vi "tcp_test.vi"() -> ()   [LabVIEW 2019]
panel:
  out "String 3":string
  in  "Numeric 2":i32=7001
  in  "String 2":string="127.0.0.1"
  in  "String":string
  out "Numeric":dbl
  in  "Boolean":bool
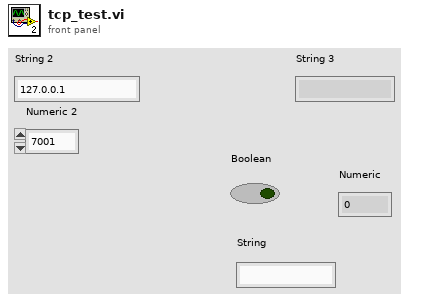
[diagram p1: front panel]
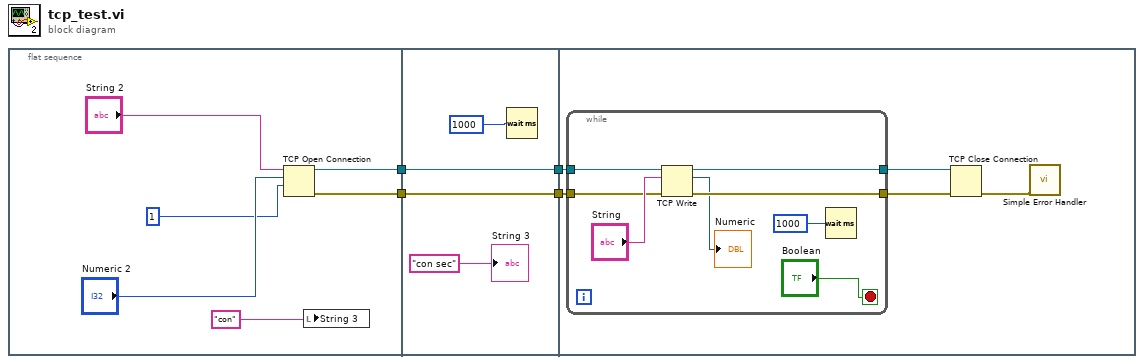
[diagram p0: block diagram]
diagram:
  n1 = flat-sequence {
    tunnel: [w8] -> w2
    tunnel: [w7] -> w1
    tunnel: [w14] -> w4
    tunnel: [w13] -> w3
    tunnel: w2 -> [w14]
    tunnel: w1 -> [w13]
    tunnel: w4 -> [w19]
    tunnel: w3 -> [w18]
    frame #0 {
      n2 = TCP Open Connection(address="String 2", remote port or service name="Numeric 2", timeout ms (60000)=1) -> (connection ID=w8:refnum<k5>, error out=w7:errorcluster)  [unwired: 2 in]
      n3 = local write "String 3"("con") -> ()
    }
    frame #1 {
      n4 = Wait (ms)(milliseconds to wait=1000) -> ()  [unwired: 1 out]
      "String 3" <- "con sec"
    }
    frame #2 {
      n5 = while {
        tunnel: w19 -> [w26]
        tunnel: w18 -> [w21]
        tunnel: [w25] -> w17
        tunnel: [w24] -> w16
        stop <- "Boolean" stop-if-true
        n6 = TCP Write(connection ID=w26, data in="String", error in (no error)=w21) -> (connection ID out=w25:refnum<k5>, bytes written=→"Numeric":i32, error out=w24:errorcluster)  [unwired: 1 in]
        n7 = Wait (ms)(milliseconds to wait=1000) -> ()  [unwired: 1 out]
      }
      n8 = TCP Close Connection(connection ID=w17, error in (no error)=w16) -> (error out=w15:errorcluster)  [unwired: 1 in, 1 out]
      n9 = call <vilib>:"Simple Error Handler.vi"("error in (no error)"=w15) -> ()  [unwired: 4 in, 5 out]
    }
  }
